vi "TwoIncoming OneOutgoing.vi"() -> ()   [LabVIEW 2015]
uses:
  <vilib>/rvi/Emulation/niFpgaGetClockAttributes.vi
  <vilib>/rvi/Emulation/niFpgaSctlEmulationGetInTimedLoop.vi
  <vilib>/rvi/Emulation/niFpgaEmulationReportErrorSimple.vi
  <vilib>/rvi/Emulation/niFpgaCriticalErrorInLSC.vi
  <vilib>/rvi/interface/RandomDataEmulation/niFpgaRandomDataHandleErrors.vi
  <vilib>/rvi/DataTransferAndStorage/Container/XNode/niFpgaContainer.xnode
  <vilib>/rvi/interface/RandomDataEmulation/nirviRandomDataFpgaReadWriteTemplate.vi
panel:
  out "Medium TO?":bool
  out "Loopback timeout":bool
  out "I16 out":i16
  out "I8 out":i8
  out "I64 out":i64
  out "I32 out":i32
  out "U16 out":u16
  out "U8 out":u8
  out "U64 out":u64
  out "U32 out":u32
  out "SGL out":sgl=2.0
  out "Boolean out":bool
  in  "Boolean":bool
  in  "SGL":sgl=1.0
  in  "U32":u32
  in  "U64":u64
  in  "U8":u8
  in  "U16":u16
  in  "I32":i32
  in  "I64":i64
  in  "I8":i8
  in  "I16":i16
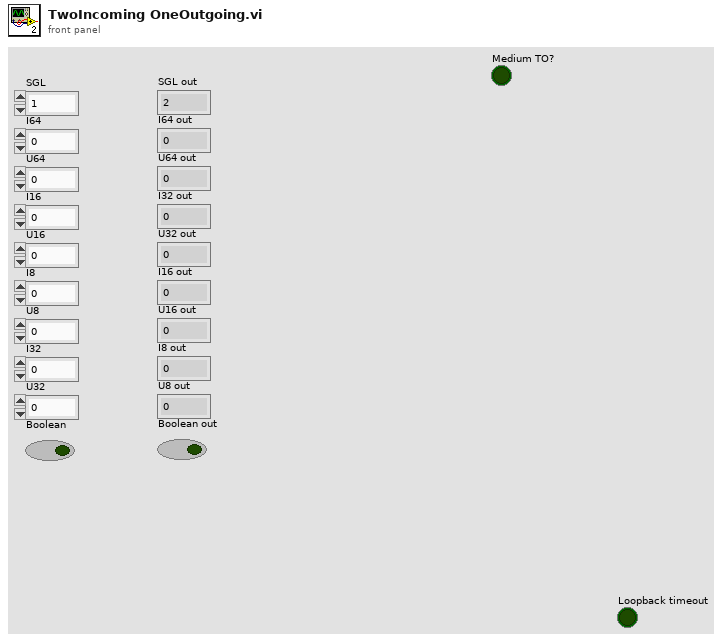
[diagram p1: front panel]
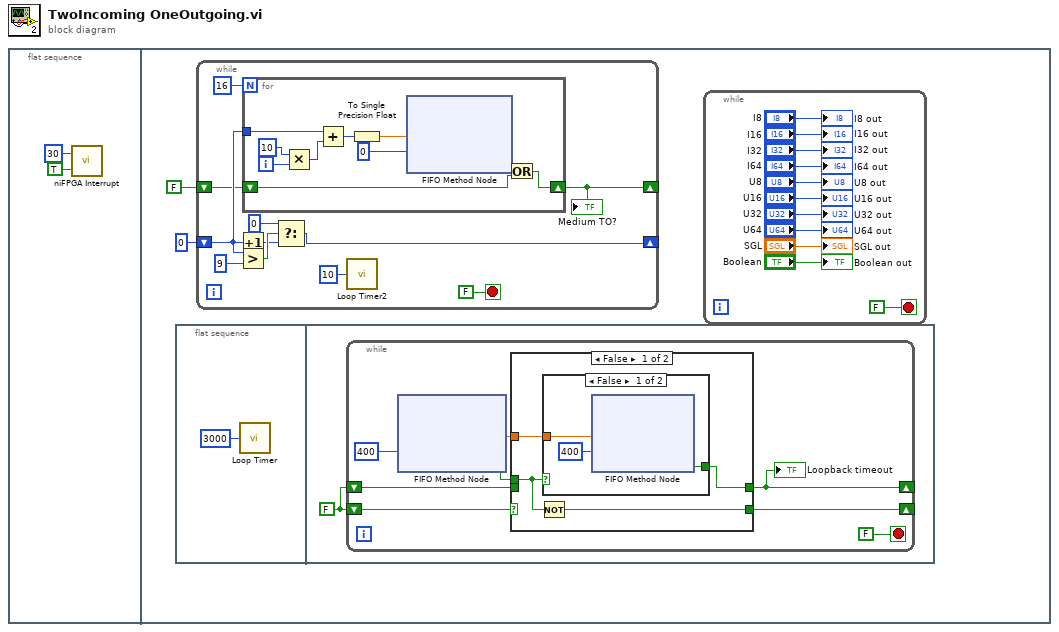
[diagram p0: block diagram]
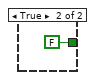
[diagram p2: hidden frame]
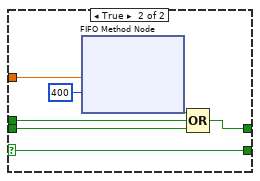
[diagram p3: hidden frame]
diagram:
  n1 = flat-sequence {
    frame #0 {
      n2 = call <vilib>:"niFPGA Interrupt.vi"("Wait Until Cleared (F)"=TRUE, "IRQ Number (0)"=u8 30) -> ()  [unwired: 1 in]
    }
    frame #1 {
      n3 = flat-sequence {
        frame #0 {
          n4 = call "Loop Timer"("Count(mSec)"=u32 3000 ("Count(uSec)")) -> ()  [unwired: 1 out]
        }
        frame #1 {
          w6 = FALSE
          n5 = while {
            shift-right: [w10] -> _
            shift-left: w6 -> [w11]
            shift-right: [w9] -> _
            shift-left: w6 -> [w8]
            stop <- FALSE stop-if-true
            n6 = xnode ("FIFO Method Node")("Timeout"=400) -> ("Element"=w12:sgl, "Timed Out?"=w7:bool)  [unwired: 1 in, 1 out]
            n7 = case shown="False" w11 {
              selector: w11 -> [_ w27]
              tunnel: w12 -> [w18 w28]
              tunnel: w7 -> [w17 w25]
              tunnel: [w16 w27] -> w10
              tunnel: [w15 w24] -> w9
              tunnel: w8 -> [_ w23]
              frame False {
                n8 = Not(x=w17) -> (.not. x?=w16:bool)
                n9 = case shown="False" w17 {
                  tunnel: w18 -> [w21 _]
                  tunnel: [w19 FALSE ("Timed Out?")] -> w15
                  frame False {
                    n10 = xnode ("FIFO Method Node")("Element"=w21, "Timeout"=400) -> ("Timed Out?"=w19:bool)  [unwired: 1 in, 1 out]
                  }
                  frame True {
                  }
                }
              }
              frame True {
                n11 = xnode ("FIFO Method Node")("Element"=w28, "Timeout"=400) -> ("Timed Out?"=w26:bool)  [unwired: 1 in, 1 out]
                n12 = Compound Arithmetic op=OR(w26, w25, w23) -> (w24:bool)
              }
            }
            "Loopback timeout" <- w9
          }
        }
      }
      n13 = while {
        shift-right: [w34] -> _
        shift-left: 0 ("t") -> [w36]
        shift-right: [w30] -> _
        shift-left: FALSE -> [w31]
        stop <- FALSE stop-if-true
        n14 = Increment(x=w36) -> (x+1=w32:i32)
        n15 = Greater?(x=w36, y=9) -> (0:w39:bool)
        n16 = for {
          N: 16 -> [_]
          tunnel: w36 -> [w50]
          shift-right: [w41] -> w30
          shift-left: w31 -> [w42]
          i -> [w49]
          n17 = Multiply(x=10, y=w49) -> (x*y=w47:i32)
          n18 = Add(x=w50, y=w47) -> (x+y=w46:i32)
          n19 = To Single Precision Float(number=w46) -> (single precision float=w45:sgl)
          n20 = xnode ("FIFO Method Node")("Element"=w45, "Timeout"=0) -> ("Timed Out?"=w43:bool)  [unwired: 1 in, 1 out]
          n21 = Or(x=w43, y=w42) -> (x .or. y?=w41:bool)
        }
        "Medium TO?" <- w30
        n22 = Select(t=0, s=w39, f=w32) -> (s? t:f=w34:i32)
        n23 = call "Loop Timer2"("Count(uSec)"=u32 10) -> ()  [unwired: 1 out]
      }
      n24 = while {
        stop <- FALSE stop-if-true
        "I16 out" <- "I16"
        "I8 out" <- "I8"
        "I64 out" <- "I64"
        "I32 out" <- "I32"
        "U16 out" <- "U16"
        "U8 out" <- "U8"
        "U64 out" <- "U64"
        "U32 out" <- "U32"
        "SGL out" <- "SGL"
        "Boolean out" <- "Boolean"
      }
    }
  }
